vi "Gen - Decimal Place (FGV).vi"(7 "Action":T1=enum."Write", 8 "error In":errorcluster, 10 "Ch2":u8, 11 "Ch1":u8) -> (0 "error out":errorcluster, 2 "Ch2 out":u8, 3 "Ch1 out":u8)   [LabVIEW 2019]
uses:
  Controls/FGV States.ctl
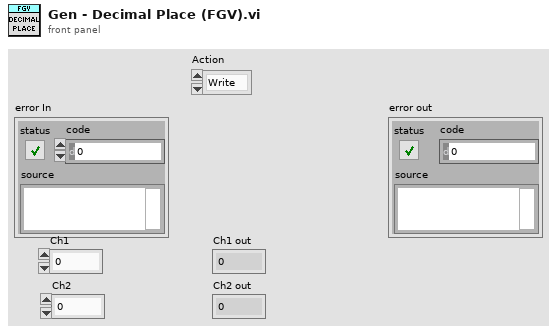
[diagram p1: front panel]
types:
  T1 = typedef "FGV States.ctl" = enum16{"Read", "Write"}
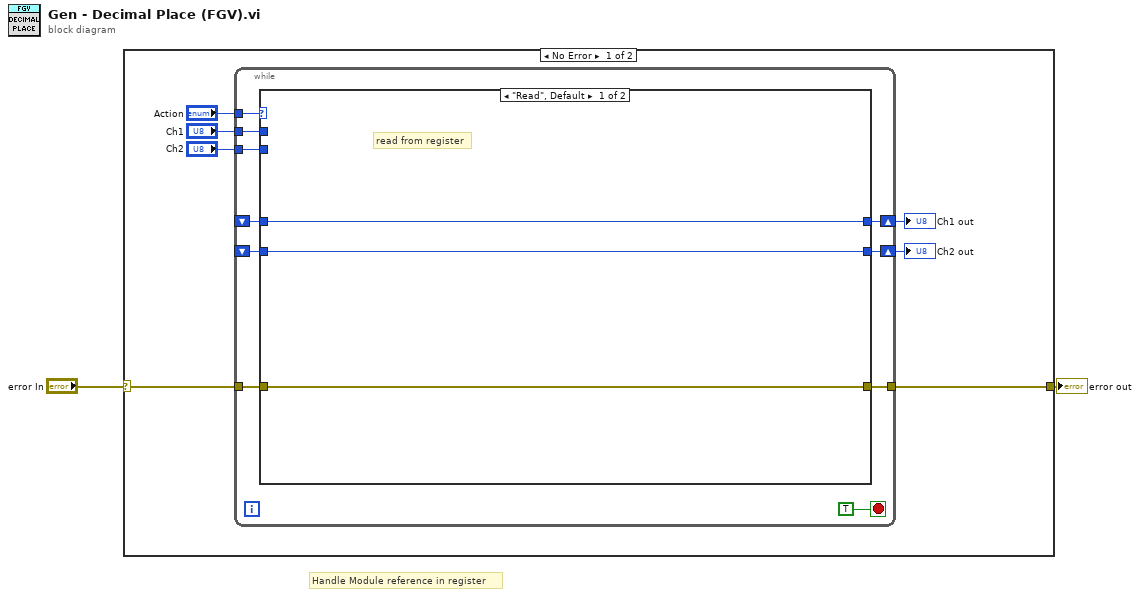
[diagram p0: block diagram]
diagram:
  # "Handle Module reference in register"
  n1 = case shown="No Error" "error In" {
    selector: "error In" -> [w8 w26]
    tunnel: [w7 w26] -> w1
    frame No Error {
      n2 = while {
        tunnel: "Action" -> [w19]
        tunnel: "Ch1" -> [w16]
        shift-right: [w17] -> w5
        shift-left: _ -> [w15]
        tunnel: [w14] -> w7
        tunnel: w8 -> [w13]
        tunnel: "Ch2" -> [w12]
        shift-right: [w11] -> w3
        shift-left: _ -> [w10]
        stop <- TRUE stop-if-true
        n3 = case shown="\"Read\", Default" w19 {
          tunnel: [w22 w25] -> w17
          tunnel: w16 -> [_ w25]
          tunnel: w15 -> [w22 _]
          tunnel: [w21 w24] -> w14
          tunnel: w13 -> [w21 w24]
          tunnel: w12 -> [_ w23]
          tunnel: [w20 w23] -> w11
          tunnel: w10 -> [w20 _]
          frame "Read", Default {
            # "read from register"
          }
          frame "Write" {
            # "write to register"
          }
        }
      }
      "Ch1 out" <- w5
      "Ch2 out" <- w3
    }
    frame Error {
    }
  }
  "error out" <- w1
